vi "publish -- glue -- number.vi"(7 "publisher action":T1, 9 "response in":refnum<user-event>, 11 "Numeric":dbl format="%#_13g") -> (0 "request event":refnum<user-event>, 1 "response out":refnum<user-event>, 3 "Numeric out":dbl)   [LabVIEW 2018]
uses:
  publisher action.ctl
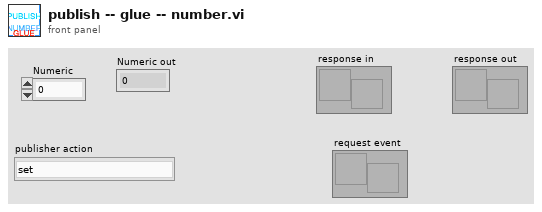
[diagram p1: front panel]
types:
  T1 = typedef "publisher action.ctl" = enum16{"set", "get", "init", "check"}
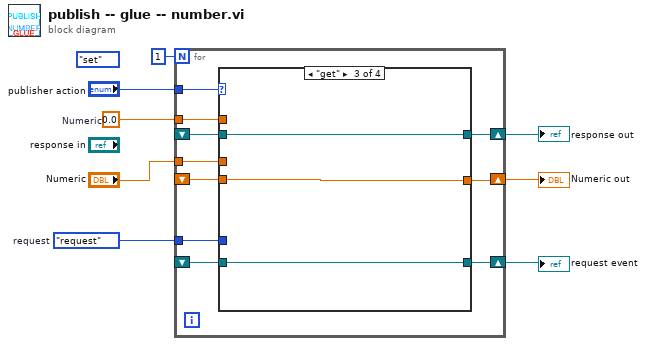
[diagram p0: block diagram]
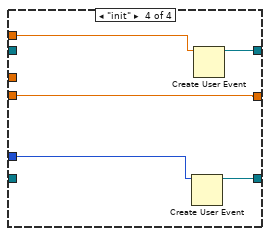
[diagram p4: hidden frame]
diagram:
  w2 = 0.0  # Numeric
  w5 = enum16{"request"}."request"  # request
  (unwired) publisher_action."set" ("publisher action")
  n1 = for {
    N: 1 -> [_]
    shift-right: [w18] -> w8
    shift-left: _ -> [w14]
    shift-right: [w17] -> w1
    shift-left: _ -> [w15]
    tunnel: "publisher action" -> [w16]
    tunnel: w2 -> [w13]
    tunnel: w5 -> [w12]
    tunnel: "Numeric" -> [w10]
    shift-right: [w11] -> w3
    shift-left: _ -> [w9]
    n2 = case shown="\"get\"" w16 {
      tunnel: [w20 w23 w26 w32] -> w18
      tunnel: [w21 w24 w27 w29] -> w17
      tunnel: w15 -> [w21 w24 w27 _]
      tunnel: w14 -> [w20 w23 w26 _]
      tunnel: w13 -> [_ _ _ w31]
      tunnel: w12 -> [_ _ _ w30]
      tunnel: [w19 w22 w25 w28] -> w11
      tunnel: w10 -> [_ w22 _ _]
      tunnel: w9 -> [w19 _ w25 w28]
      frame "check", Default {
      }
      frame "set" {
      }
      frame "get" {
      }
      frame "init" {
        n3 = Create User Event(user event datatype=w30) -> (user event=w32:refnum<user-event>)  [unwired: 1 in, 1 out]
        n4 = Create User Event(user event datatype=w31) -> (user event=w29:refnum<user-event>)  [unwired: 1 in, 1 out]
      }
    }
  }
  "request event" <- w8
  "Numeric out" <- w3
  "response out" <- w1
